vi "compare readings NANOVNA.vi"() -> ()   [LabVIEW 2020]
uses:
  common/record_file_handler/VFH-VNA_File_Handler.lvlib
  common/features/CF-common_features.lvlib
panel:
  out "Array 4":errorcluster[](array[cluster])
  out "Array 3":bool[](array[boolean])
  out "Array 2":path[](array[path])
  out "S11 I":cluster{"Frequency":dbl[], "S21_Imag":dbl[]}[](graph)
  out "Magnitude":cluster{"Frequency":dbl[], "S21_Imag":dbl[]}[](graph)
  out "|Z|":cluster{"Frequency":dbl[], "S21_Imag":dbl[]}[](graph)
  out "S11 R":cluster{"Frequency":dbl[], "S21_Imag":dbl[]}[](graph)
  in  "Signal":i32
  out "Cluster":T1 {"Z''" format="%#_5p"; "Z'" format="%#_5p"; "|Z|" format="%#_5p"; "Loss" format="%#_5p"; "Deg" format="%#_5p"; "Phi" format="%#_5p"; "Mag" format="%#_5p"; "S11 I" format="%#_5p"; "S11 R" format="%#_5p"}
  out "Array":dbl[](array[numeric]) format="%#_5p"
  out "Freq":dbl format="%#_6p"
  in  "index":i32
  in  "Stop":bool
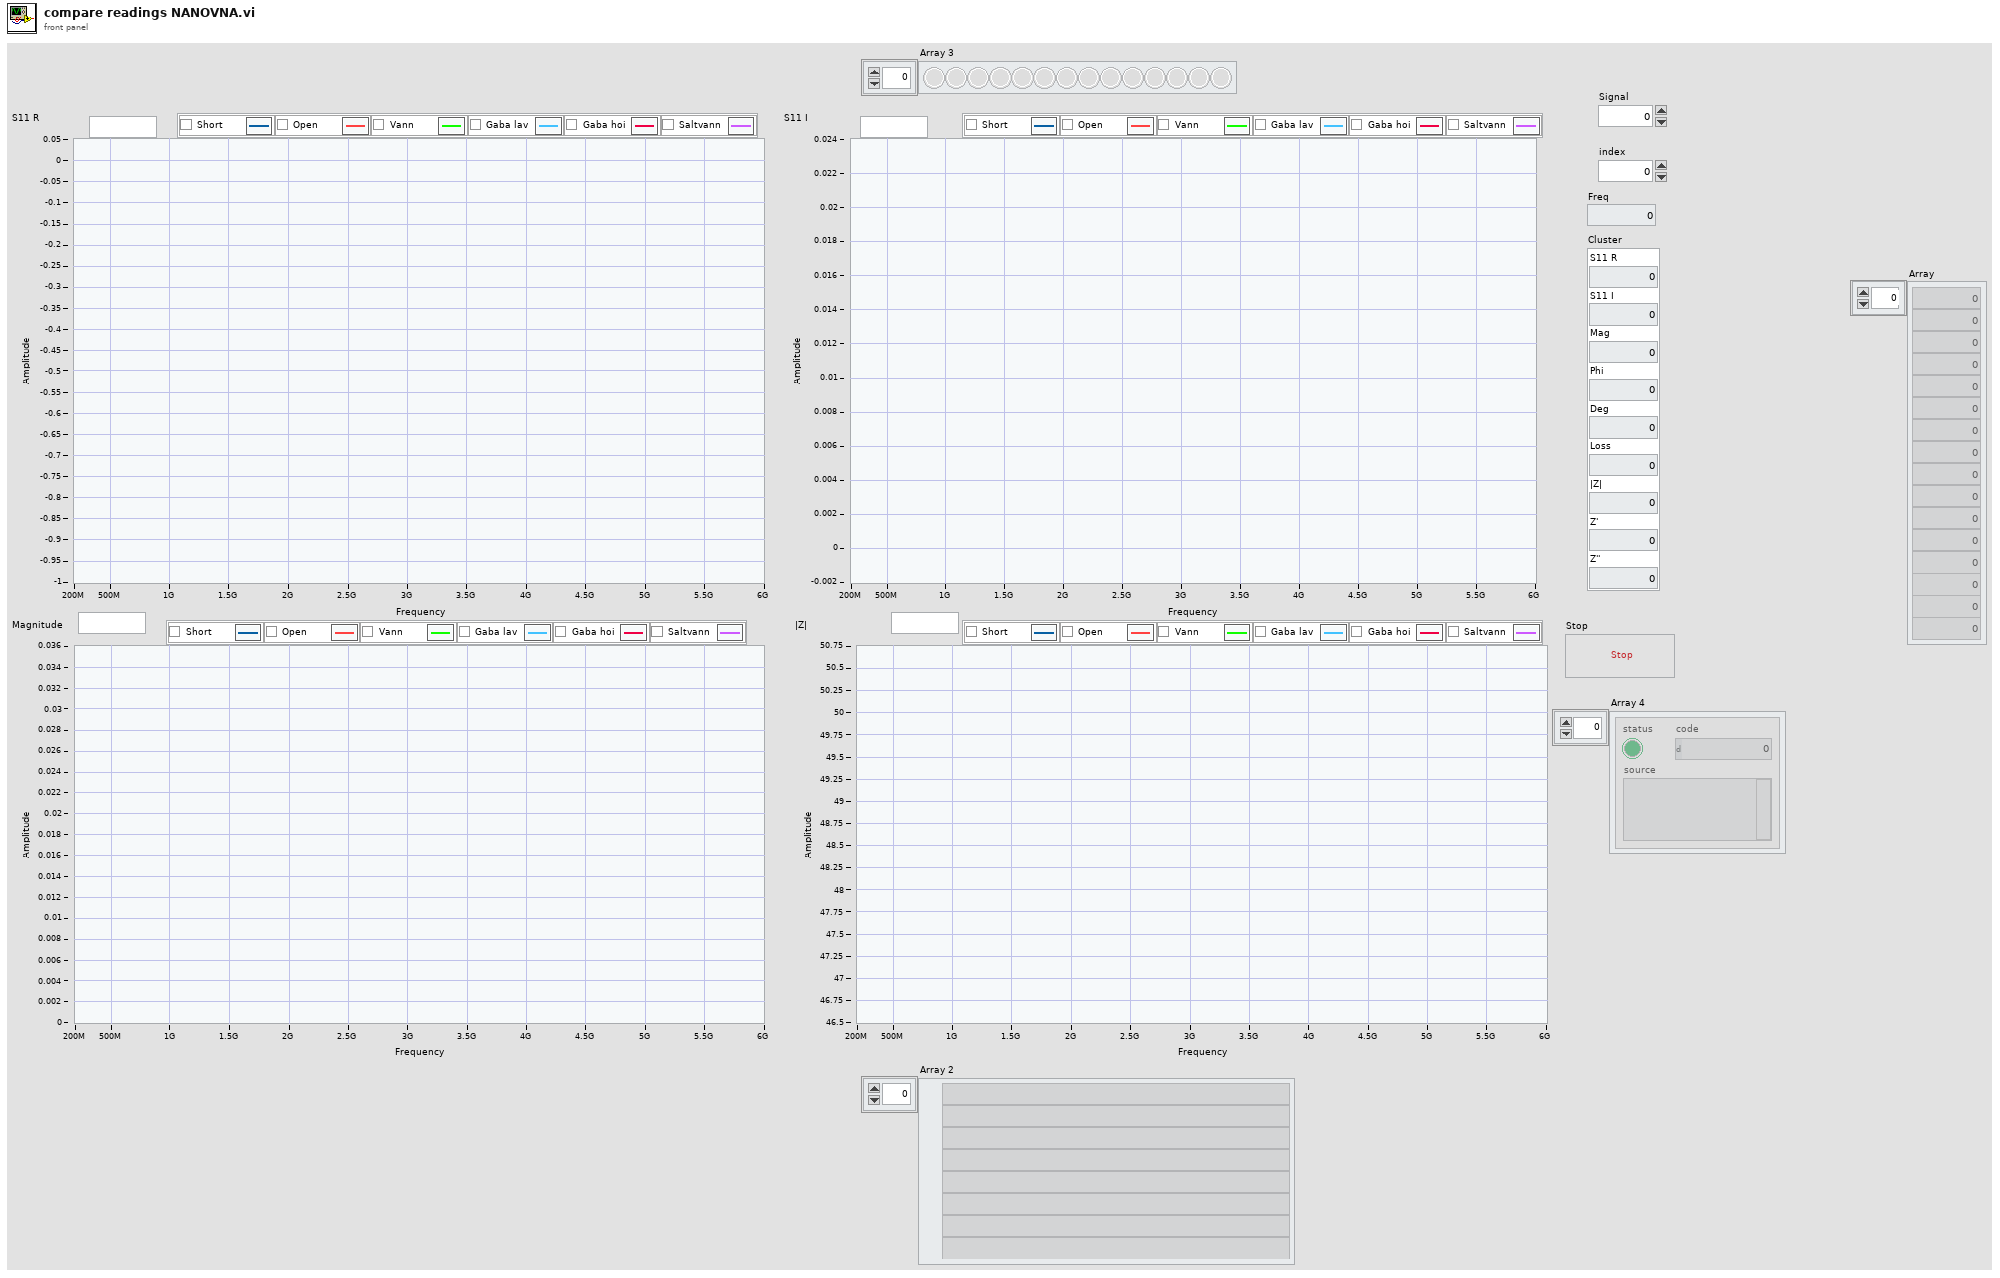
[diagram p1: front panel]
types:
  T1 = cluster{"S11 R":dbl, "S11 I":dbl, "Mag":dbl, "Phi":dbl, "Deg":dbl, "Loss":dbl, "|Z|":dbl, "Z'":dbl, "Z''":dbl}
  T2 = typedef "VFH-VNA_File_Handler.lvlib/VFH-file_cluster-NanoVNA.ctl" = cluster{"Frequency":dbl[], "S11_Real":dbl[], "S11_Imag":dbl[], "S21_Real":dbl[], "S21_Imag":dbl[], "S12_Real":dbl[], "S12_Imag":dbl[], "S22_Real":dbl[], "S22_Imag":dbl[]}
  T3 = cluster{"Loss":cluster{"Frequency":dbl[], "Array":dbl[]}, "Z Modulus":cluster{"Frequency":dbl[], "Array":dbl[]}, "Z'":cluster{"Frequency":dbl[], "Array":dbl[]}, "Z''":cluster{"Frequency":dbl[], "Array":dbl[]}}
  T4 = cluster{"S11'":cluster{"Frequency":dbl[], "S11_Real":dbl[]}, "S11''":cluster{"Frequency":dbl[], "S11_Real":dbl[]}, "Magnitude":cluster{"Frequency":dbl[], "Array":dbl[]}, "Eta":cluster{"Frequency":dbl[], "Array":dbl[]}, "Phase":cluster{"Frequency":dbl[], "Array":dbl[]}}
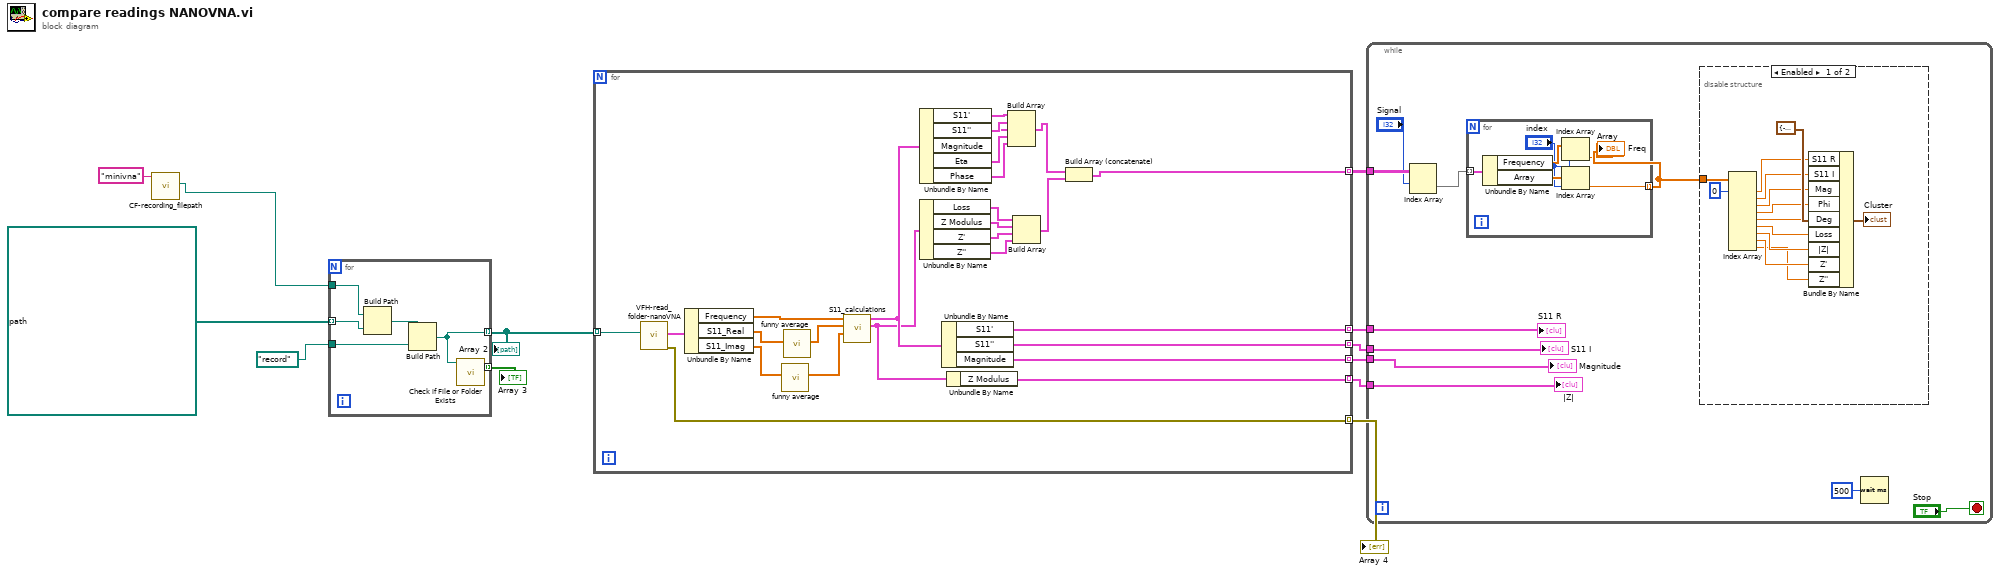
[diagram p0: block diagram]
diagram:
  n1 = call "CF-recording_filepath.vi"("Input path"="minivna") -> ("data Path + input"=w1:path)  [unwired: 9 in, 1 out]
  n2 = for {
    tunnel: path[] [path "test-short", path "test-open", path "test-Vann", path "test-Gabalav", path "test-gabahøy", path "test-Saltvann"] ("Folder Path") -> [w17] mode=indexing
    tunnel: w1 -> [w18]
    tunnel: [w14] -> w6 mode=indexing
    tunnel: [w16] -> w5 mode=indexing
    tunnel: path "record" ("name or relative path") -> [w13]
    n3 = Build Path(base path=w18, name or relative path=w17) -> (appended path=w15:path)
    n4 = Build Path(base path=w15, name or relative path=w13) -> (appended path=w14:path)
    n5 = call <vilib>:"Check if File or Folder Exists.vi"("path"=w14) -> ("file or folder exists?"=w16:bool)  [unwired: 8 in, 2 out]
  }
  "Array 2" <- w6
  "Array 3" <- w5
  n6 = for {
    tunnel: w6 -> [w30] mode=indexing
    tunnel: [w28] -> w12 mode=indexing
    tunnel: [w27] -> w11 mode=indexing
    tunnel: [w26] -> w9 mode=indexing
    tunnel: [w25] -> w10 mode=indexing
    tunnel: [w24] -> w8 mode=indexing
    tunnel: [w19] -> w3 mode=indexing
    n7 = call "VFH-read_folder-nanoVNA.vi"("Folder Path"=w30) -> ("error out"=w19:errorcluster, "avg output"=w29:T2)  [unwired: 7 in, 2 out]
    n8 = Unbundle By Name(w29) -> ("Frequency"=w44:dbl[], "S11_Real"=w23:dbl[], "S11_Imag"=w21:dbl[])
    n9 = call "funny average.vi"("in"=w21) -> ("Out"=w20:dbl[])  [unwired: 10 in]
    n10 = call "funny average.vi"("in"=w23) -> ("Out"=w22:dbl[])  [unwired: 10 in]
    n11 = call "S11_calculations.vi"("S11_Imag"=w20, "S11_Real"=w22, "Frequency"=w44) -> ("Calc"=w31:T3, "Raw"=w32:T4)  [unwired: 6 in, 1 out]
    n12 = Unbundle By Name(w32) -> ("S11'"=w43:cluster{"Frequency":dbl[], "S11_Real":dbl[]}, "S11''"=w42:cluster{"Frequency":dbl[], "S11_Real":dbl[]}, "Magnitude"=w41:cluster{"Frequency":dbl[], "Array":dbl[]}, "Eta"=w40:cluster{"Frequency":dbl[], "Array":dbl[]}, "Phase"=w39:cluster{"Frequency":dbl[], "Array":dbl[]})
    n13 = Unbundle By Name(w31) -> ("Loss"=w38:cluster{"Frequency":dbl[], "Array":dbl[]}, "Z Modulus"=w37:cluster{"Frequency":dbl[], "Array":dbl[]}, "Z'"=w36:cluster{"Frequency":dbl[], "Array":dbl[]}, "Z''"=w35:cluster{"Frequency":dbl[], "Array":dbl[]})
    n14 = Unbundle By Name(w32) -> ("S11'"=w28:cluster{"Frequency":dbl[], "S11_Real":dbl[]}, "S11''"=w27:cluster{"Frequency":dbl[], "S11_Real":dbl[]}, "Magnitude"=w26:cluster{"Frequency":dbl[], "Array":dbl[]})
    n15 = Unbundle By Name(w31) -> ("Z Modulus"=w25:cluster{"Frequency":dbl[], "Array":dbl[]})
    n16 = Build Array(w43, w42, w41, w40, w39) -> (w33:cluster{"Frequency":dbl[], "Array":dbl[]}[])
    n17 = Build Array(w38, w37, w36, w35) -> (w34:cluster{"Frequency":dbl[], "Array":dbl[]}[])
    n18 = Build Array (concatenate)(w33, w34) -> (w24:cluster{"Frequency":dbl[], "Array":dbl[]}[])
  }
  "Array 4" <- w3
  n19 = while {
    tunnel: w12 -> [w54]
    tunnel: w11 -> [w53]
    tunnel: w10 -> [w52]
    tunnel: w9 -> [w51]
    tunnel: w8 -> [w49]
    stop <- "Stop" stop-if-true
    n20 = Index Array(array=w49, index (row)="Signal") -> (element=w48:cluster{"Frequency":dbl[], "Array":dbl[]}[])  [unwired: 1 in]
    n21 = for {
      tunnel: w48 -> [w60] mode=indexing
      tunnel: [w55] -> w50 mode=indexing
      n22 = Unbundle By Name(w60) -> ("Frequency"=w58:dbl[], "Array"=w59:dbl[])
      n23 = Index Array(array=w58, index="index") -> (element=→"Freq":dbl)
      n24 = Index Array(array=w59, index="index") -> (element=w55:dbl)
    }
    "Array" <- w50
    n25 = disable-structure shown="Enabled" {
      disable-tunnel: w50 -> [w73 _]
      frame Enabled {
        n26 = Index Array(array=w73, index #1=0 ("index (row)")) -> (element #1=w70:dbl, element #2=w69:dbl, element #3=w68:dbl, element #4=w67:dbl, element #5=w66:dbl, element #6=w65:dbl, element #7=w64:dbl, element #8=w63:dbl, element #9=w62:dbl)  [unwired: 8 in]
        n27 = Bundle By Name(cluster=T1 {"S11 R"=-0.13079270605384616, "S11 I"=-0.13079270605384616, "Mag"=-0.13079270605384616, "Phi"=-0.13079270605384616, "Deg"=-0.13079270605384616, "Loss"=-0.13079270605384616, "|Z|"=-0.13079270605384616, "Z'"=-0.13079270605384616, "Z''"=-0.13079270605384616} ("Cluster"), "S11 R"=w70, "S11 I"=w69, "Mag"=w68, "Phi"=w67, "Deg"=w66, "Loss"=w65, "|Z|"=w64, "Z'"=w63, "Z''"=w62) -> (→"Cluster":T1)
      }
      frame Disabled {
      }
    }
    n28 = Wait (ms)(milliseconds to wait=u32 500) -> ()  [unwired: 1 out]
    "Magnitude" <- w51
    "S11 R" <- w54
    "|Z|" <- w52
    "S11 I" <- w53
  }
